vi "rtlsdr_read_to_waveform.vi"(6 "timestamp index":dbl, 7 "ref in":refnum<k5>, 8 "error in (no error)":errorcluster, 9 "buffer size":i32=1024, 10 "sample rate":i32=1024) -> (0 "error out":errorcluster, 1 "output downconverted waveform":cluster{dbl, dbl, cdb[]}, 2 "output waveform":waveform(cdb), 3 "output array":cdb[](array[numeric]), 4 "next timestamp index":dbl, 5 "ref out":refnum<k5>)   [LabVIEW 2011]
panel:
  # "Outputs:"
  # "Inputs:"
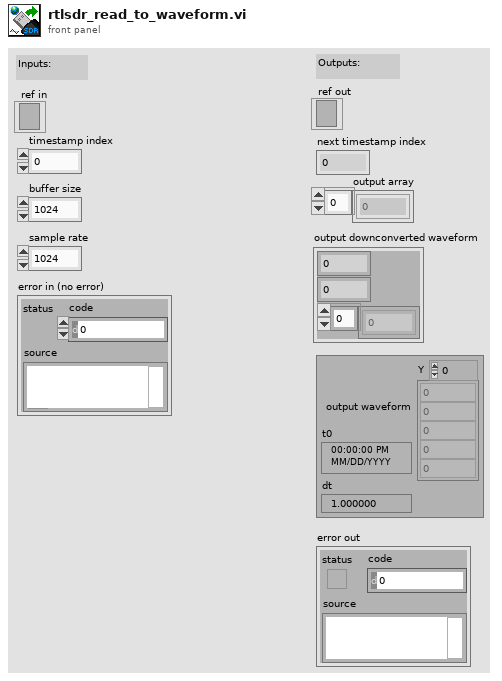
[diagram p1: front panel]
types:
  T1 = enum16{"Standard", "Buffered", "CRLF", "Immediate"}
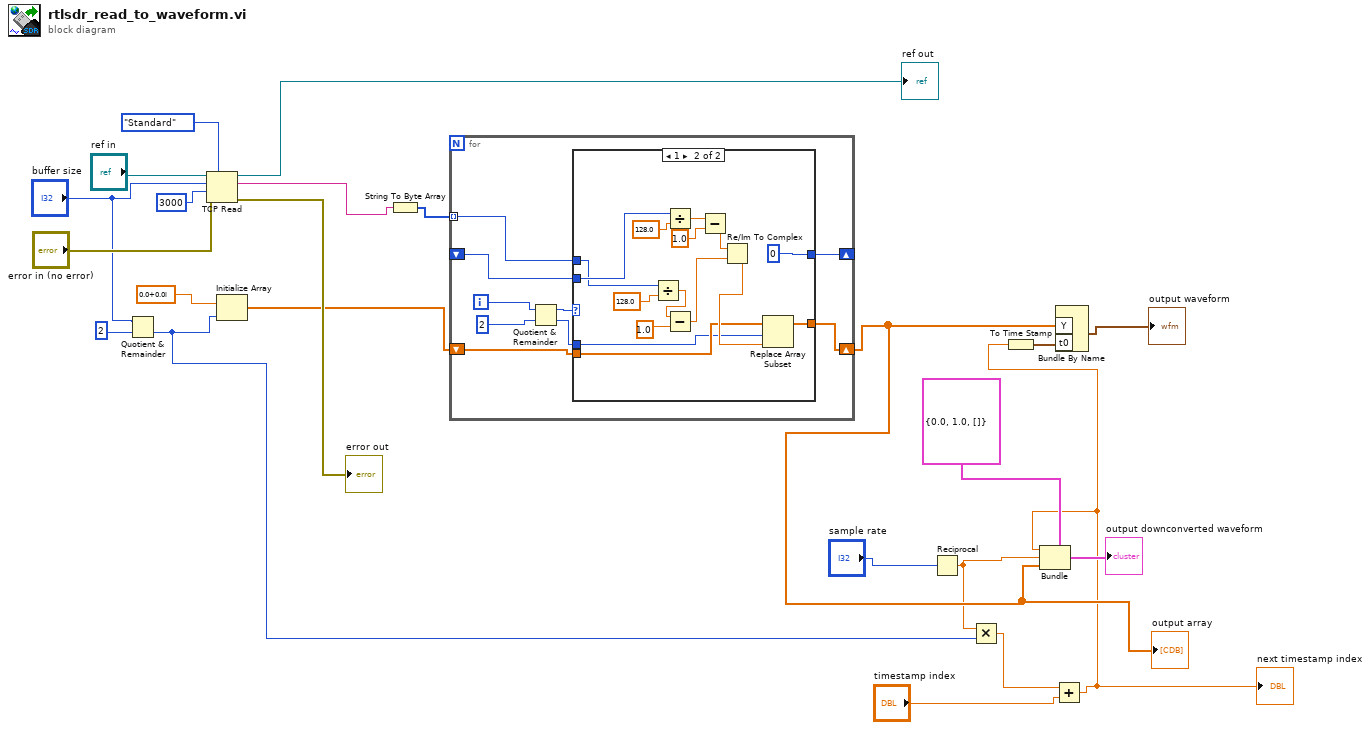
[diagram p0: block diagram]
diagram:
  n1 = Quotient & Remainder(x="buffer size", y=2) -> (floor(x/y)=w1:i32)  [unwired: 1 out]
  n2 = TCP Read(connection ID="ref in", bytes to read="buffer size", error in (no error)="error in (no error)", 7:T1."Standard" ("mode (standard)"), 9:3000 ("timeout ms (25000)")) -> (connection ID out=→"ref out":refnum<k5>, data out=w19:string, error out=→"error out":errorcluster)
  n3 = Initialize Array(cdb 0.0+0.0i ("element"), w1) -> (w13:cdb[])
  n4 = String To Byte Array(string=w19) -> (unsigned byte array=w18:u8[])
  n5 = for {
    tunnel: w18 -> [w29] mode=indexing
    shift-right: [w28] -> _
    shift-left: _ -> [w27]
    shift-right: [w24] -> w9
    shift-left: w13 -> [w26]
    i -> [w32]
    n6 = Quotient & Remainder(x=w32, y=2) -> (x-y*floor(x/y)=w30:i32, floor(x/y)=w25:i32)
    n7 = case shown="1" w30 {
      tunnel: w29 -> [w34 w47]
      tunnel: [w34 u8 0] -> w28
      tunnel: w27 -> [_ w48]
      tunnel: w26 -> [w33 w37]
      tunnel: w25 -> [_ w36]
      tunnel: [w33 w35] -> w24
      frame 0, Default {
      }
      frame 1 {
        n8 = Divide(x=w47, y=128.0) -> (x/y=w42:dbl)
        n9 = Divide(x=w48, y=128.0) -> (x/y=w44:dbl)
        n10 = Subtract(x=w42, y=1.0) -> (x-y=w40:dbl)
        n11 = Subtract(x=w44, y=1.0) -> (x-y=w39:dbl)
        n12 = Re/Im To Complex(1:w40, 2:w39) -> (0:w38:cdb)
        n13 = Replace Array Subset(array=w37, new element=w38, index=w36) -> (w35:cdb[])
      }
    }
  }
  "output array" <- w9
  n14 = Reciprocal(x="sample rate") -> (1/x=w2:dbl)
  n15 = Multiply(x=w2, y=w1) -> (x*y=w7:dbl)
  n16 = Add(x=w7, y="timestamp index") -> (x+y=w5:dbl)
  "next timestamp index" <- w5
  n17 = To Time Stamp(1:w5) -> (0:w4:timestamp)
  n18 = Bundle(cluster=cluster{dbl, dbl, cdb[]} {0.0, 1.0, []}, w5, w2, w9) -> (→"output downconverted waveform":cluster{dbl, dbl, cdb[]})
  n19 = Bundle By Name("Y"=w9, "t0"=w4) -> (→"output waveform":waveform(cdb))  [unwired: 1 in]
